vi "PQexpressCmd.vi"(8 "error in (no error)":errorcluster, 10 "Command":string, 11 "conninfo":T1={"host"="localhost", "port"="5432", "client_encoding"="WIN1251", "dbname"="data", "user"="postgres", "password"=""}) -> (0 "error out":errorcluster, 1 "DatabaseMessages":T2, 2 "column_names":string[](array[string]), 3 "data":string[][](array[string]))   [LabVIEW 2019, in "libpqutility.lvlib"]
doc: "set the connection string, type in your SQL cmd and fire! The Result Data is provided as Array of String"
uses:
  libpqutility.lvlib
  libpqlv/src/PQfinish.vi
  libpqlv/src/PQconnectdb.vi
  libpqlv/src/PQerrorMessage.vi
  libpqlv/src/PQstatus.vi
  <vilib>/dlg_ctls.llb/Space Constant.vi
  libpqlv/src/PQclear.vi
  PQsyncQueryCommand.vi
  PQfetchResultData.vi
  PQfetchColumnNames.vi
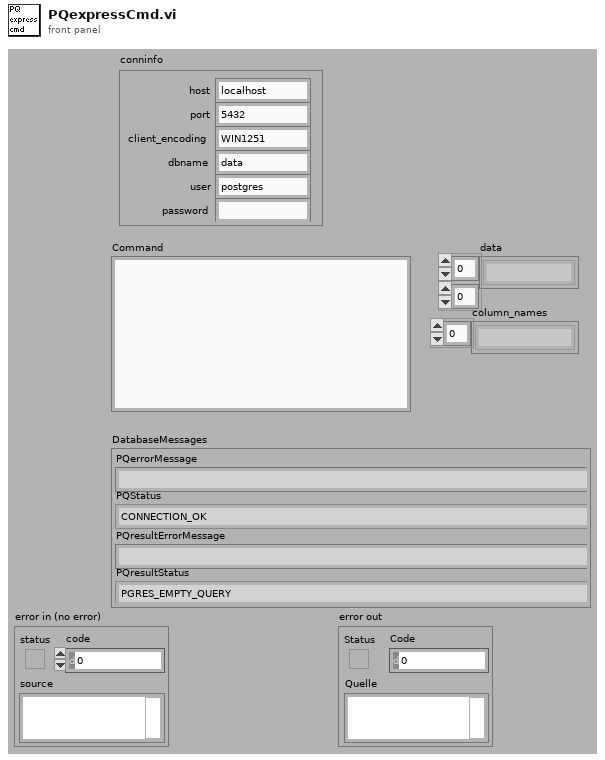
[diagram p1: front panel]
types:
  T1 = cluster{"host":string, "port":string, "client_encoding":string, "dbname":string, "user":string, "password":string}
  T2 = cluster{"PQerrorMessage":string, "PQStatus":enum16{"CONNECTION_OK", "CONNECTION_BAD", "CONNECTION_STARTED", "CONNECTION_MADE", "CONNECTION_AWAITING_RESPONSE", "CONNECTION_AUTH_OK", "CONNECTION_SETENV", "CONNECTION_SSL_STARTUP", "CONNECTION_NEEDED"}, "PQresultErrorMessage":string, "PQresultStatus":enum16{"PGRES_EMPTY_QUERY", "PGRES_COMMAND_OK", "PGRES_TUPLES_OK", "PGRES_COPY_OUT", "PGRES_COPY_IN", "PGRES_BAD_RESPONSE", "PGRES_NONFATAL_ERROR", "PGRES_FATAL_ERROR"}}
  T3 = enum32{"CONNECTION_OK", "CONNECTION_BAD", "CONNECTION_STARTED", "CONNECTION_MADE", "CONNECTION_AWAITING_RESPONSE", "CONNECTION_AUTH_OK", "CONNECTION_SETENV", "CONNECTION_SSL_STARTUP", "CONNECTION_NEEDED"}
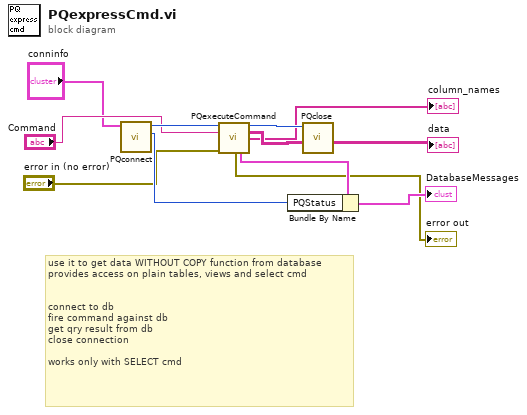
[diagram p0: block diagram]
diagram:
  # "use it to get data WITHOUT COPY function from database\nprovides access on plain tables, views and select cmd\n\n\nconnect to db\nfire command against db\nget qry result from db\nclose connection\n\nworks only with SELECT cmd"
  n1 = call "PQconnect.vi"("conninfo"="conninfo") -> ("PQStatus"=w11:T3, "conn"=w9:u32)  [unwired: 8 in, 1 out]
  n2 = call "PQexecuteCommand.vi"("conn"=w9, "Command"="Command", "error in (no error)"="error in (no error)") -> ("conn_out"=w6:u32, "Data"=→"data":string[][], "ColumnNames"=→"column_names":string[], "error out"=→"error out":errorcluster, "DatabaseMesssageCluster"=w3:T2)  [unwired: 6 in, 2 out]
  n3 = Bundle By Name(cluster=w3, "PQStatus"=w11) -> (→"DatabaseMessages":T2)
  n4 = call "PQclose.vi"("conn"=w6) -> ()  [unwired: 10 in, 1 out]
